vi "COMI US Start.vi"(5 "trsMethod":i32, 6 "msb":u32, 7 "scanFreq":u32, 9 "chanList":i32, 10 "numCh":i32, 11 "hDevice":u32) -> (2 "function return":i32, 3 "hDevice out":u32)   [LabVIEW 2017, in "Comidll.lvlib"]
doc: "long (COMI_US_Start) (HANDLE hDevice, int numCh, int chanList, unsigned int scanFreq,\n unsigned int msb, int trsMethod);"
uses:
  <userlib>/Comidll/Comidll.lvlib
  <userlib>/Comidll/Comidll.dll
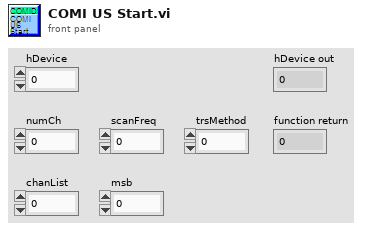
[diagram p1: front panel]
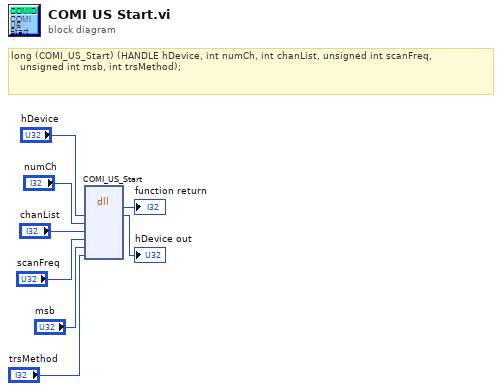
[diagram p0: block diagram]
diagram:
  # "long\t(COMI_US_Start) (HANDLE hDevice, int numCh, int chanList, unsigned int scanFreq,\n\t\t\tunsigned int msb, int trsMethod);"
  n1 = dll-call lib="C:/Program Files/National Instruments/LabVIEW 2017/user.lib/Comidll/Comidll.*" fn="COMI_US_Start"("hDevice"="hDevice", "numCh"="numCh", "chanList"="chanList", "scanFreq"="scanFreq", "msb"="msb", "trsMethod"="trsMethod") -> (→"function return":i32, "hDevice"=→"hDevice out":u32)  [unwired: 8 in, 2 out]
